vi "USB2XXXSPIADS1256.vi"() -> ()   [LabVIEW 2010]
uses:
  PublicFiles/usb_device/USB2XXX.dll
panel:
  out "mVp-p":dbl
  out "DC":dbl
  out "RMS":dbl
  out "Waveform Chart":dbl(graph)
  in  "pConfig":T1
  in  "Channel Index":i32(ring) items=["SPI1_CS0", "SPI2_CS0"]
  in  "Device Index":i32(ring) items=["0", "1", "2", "3", "4", "5"]
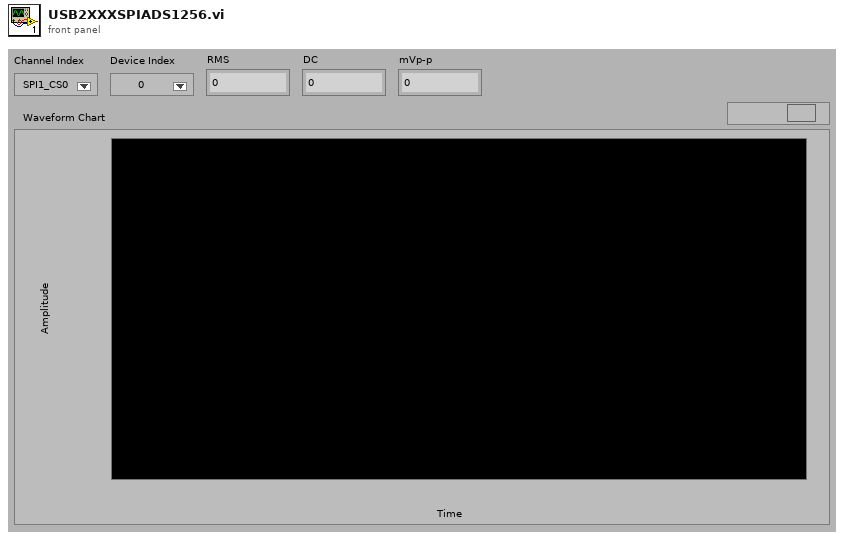
[diagram p1: front panel]
types:
  T1 = cluster{"Mode":i8, "Master":i8, "CPOL":i8, "CPHA":i8, "LSBFirst":i8, "SelPolarity":i8, "@dummy control@":i8, "@dummy control@":i8, "ClockSpeedHz":u32}
  T2 = enum16{"Init ADS1256", "Init SPI", "Read Data", "Close"}
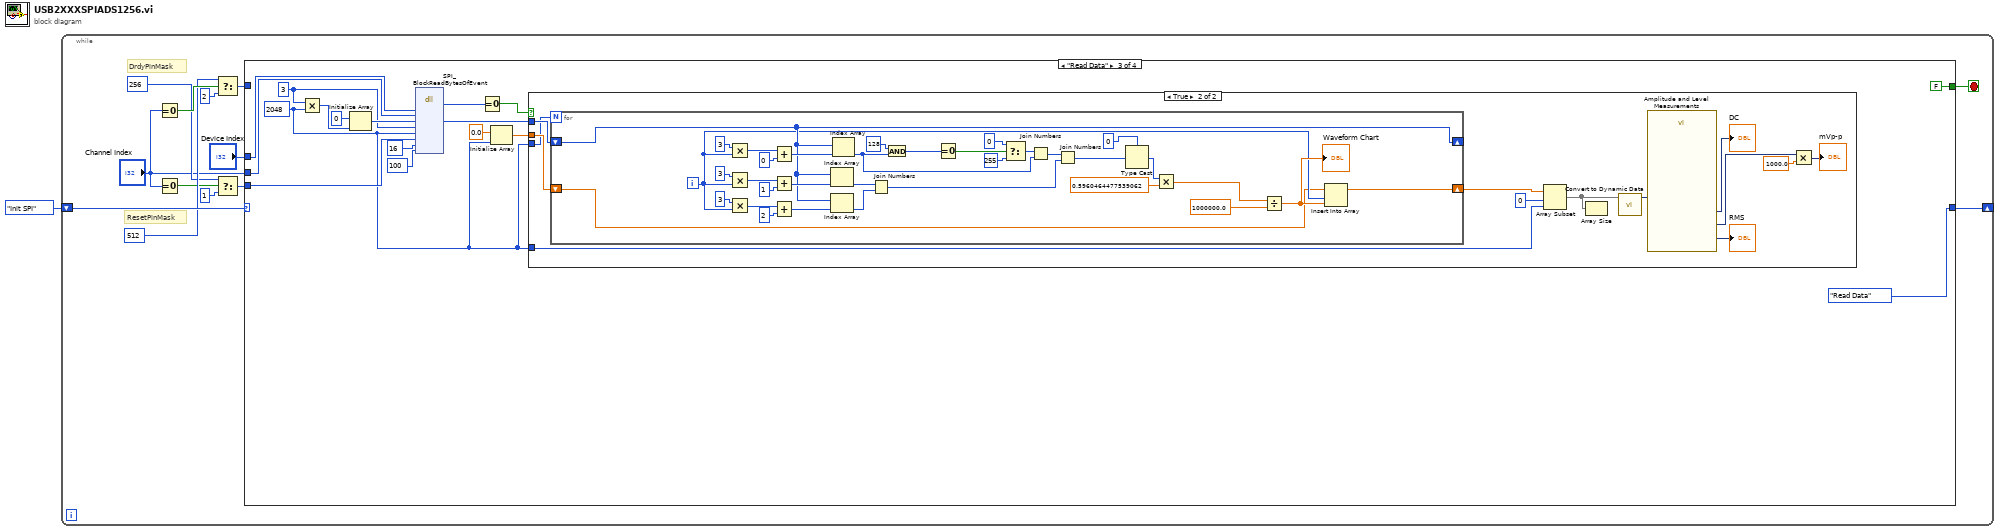
[diagram p0: block diagram]
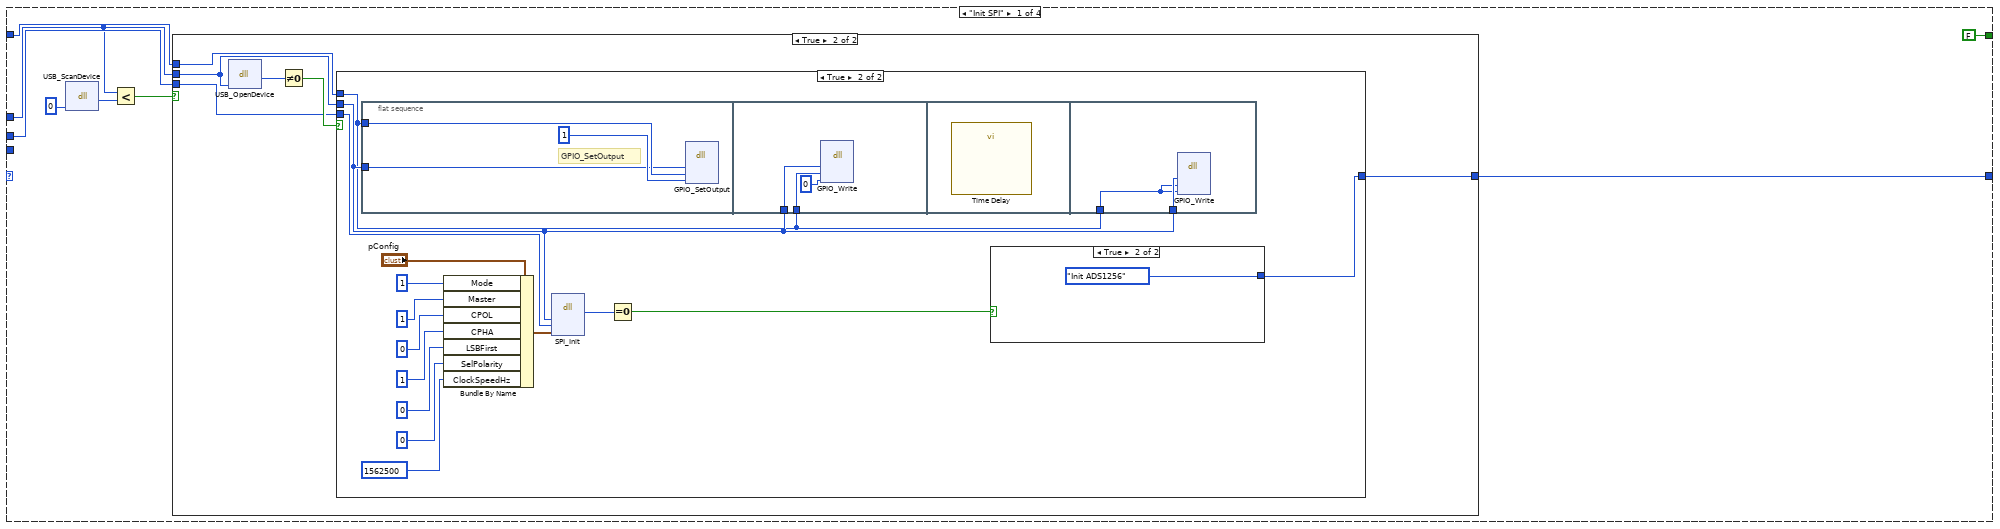
[diagram p2: hidden frame]
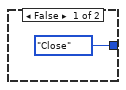
[diagram p3: hidden frame]
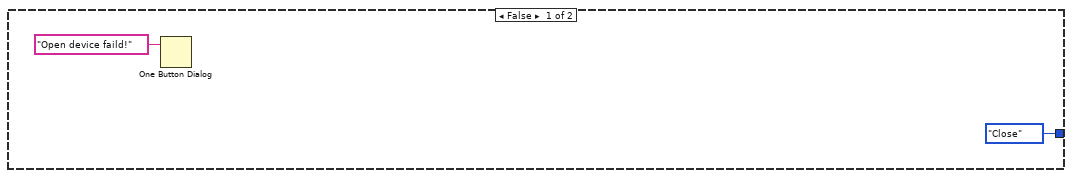
[diagram p4: hidden frame]
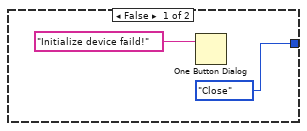
[diagram p5: hidden frame]
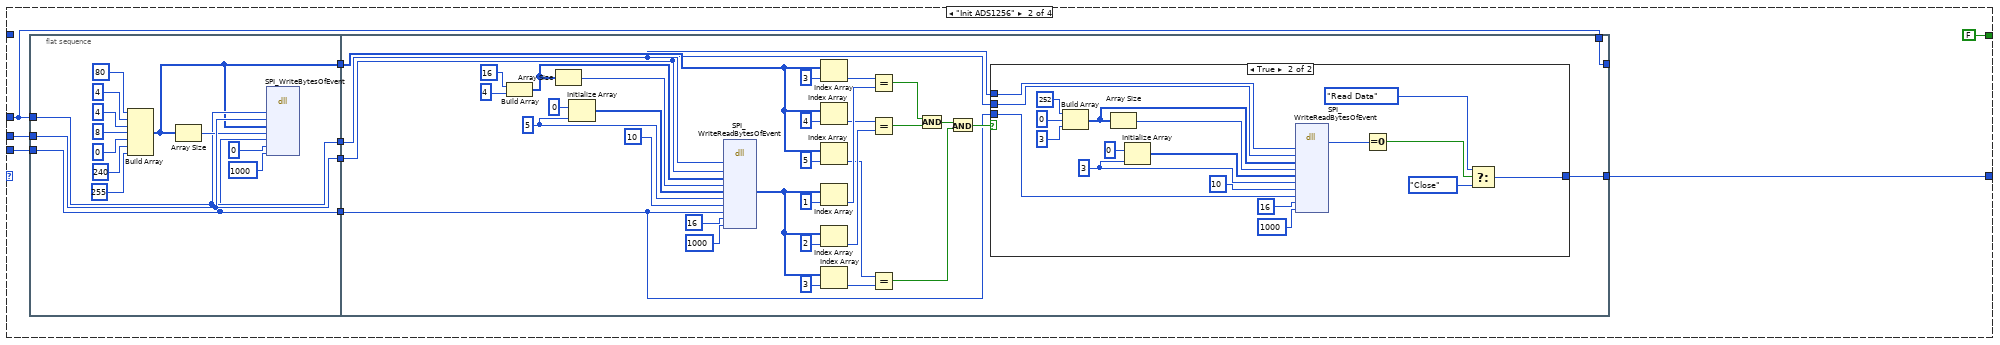
[diagram p6: hidden frame]
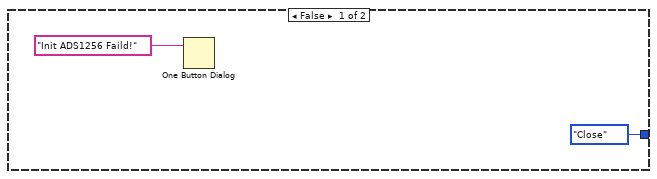
[diagram p7: hidden frame]
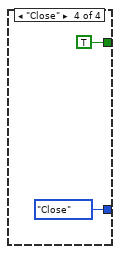
[diagram p9: hidden frame]
diagram:
  n1 = while {
    shift-right: [w13] -> _
    shift-left: T2."Init SPI" ("Enum") -> [w14]
    stop <- w11 stop-if-true
    # "DrdyPinMask"
    # "ResetPinMask"
    n2 = Equal To 0?(x="Channel Index") -> (x = 0?=w10:bool)
    n3 = Equal To 0?(x="Channel Index") -> (x = 0?=w7:bool)
    n4 = Select(t=u32 512 ("SelPolarity"), s=w10, f=u32 2 ("SelPolarity")) -> (s? t:f=w3:u32)
    n5 = Select(t=u32 256 ("SelPolarity"), s=w7, f=u32 1 ("SelPolarity")) -> (s? t:f=w2:u32)
    n6 = case shown="\"Read Data\"" w14 {
      tunnel: [w19 w58 T2."Read Data" ("Enum") T2."Close" ("Enum")] -> w13
      tunnel: "Device Index" -> [w16 w63 w149 _]
      tunnel: "Channel Index" -> [w18 w65 w148 _]
      tunnel: [FALSE FALSE FALSE TRUE] -> w11
      tunnel: w3 -> [w15 _ _ _]
      tunnel: w2 -> [_ w62 w144 _]
      frame "Init SPI" {
        n7 = dll-call lib="F:/OtherWork/STM32/USB2XXX_Example/trunk/Labview/PublicFiles/usb_device/USB2XXX.*" fn="USB_ScanDevice"("pDevNum"=0) -> (w21:i32)  [unwired: 4 in, 2 out]
        n8 = Less?(x=w16, y=w21) -> (x < y?=w20:bool)
        n9 = case shown="True" w20 {
          tunnel: w16 -> [_ w25]
          tunnel: w18 -> [_ w27]
          tunnel: [T2."Close" ("Enum") w26] -> w19
          tunnel: w15 -> [_ w24]
          frame False {
          }
          frame True {
            n10 = dll-call lib="F:/OtherWork/STM32/USB2XXX_Example/trunk/Labview/PublicFiles/usb_device/USB2XXX.*" fn="USB_OpenDevice"("DevIndex"=w25) -> (w29:u8)  [unwired: 4 in, 2 out]
            n11 = Not Equal To 0?(x=w29) -> (x != 0?=w28:bool)
            n12 = case shown="True" w28 {
              tunnel: w27 -> [_ w34]
              tunnel: w25 -> [_ w33]
              tunnel: [T2."Close" ("Enum") w45] -> w26
              tunnel: w24 -> [_ w32]
              frame False {
                n13 = One Button Dialog(message="Open device faild!") -> ()  [unwired: 1 in, 1 out]
              }
              frame True {
                n14 = flat-sequence {
                  tunnel: w32 -> [w48]
                  tunnel: w33 -> [w47]
                  tunnel: w33 -> [w52]
                  tunnel: w32 -> [w51]
                  tunnel: w33 -> [w54]
                  tunnel: w32 -> [w53]
                  frame #0 {
                    # "GPIO_SetOutput"
                    n15 = dll-call lib="F:/OtherWork/STM32/USB2XXX_Example/trunk/Labview/PublicFiles/usb_device/USB2XXX.*" fn="GPIO_SetOutput"("DevIndex"=w47, "PinMask"=w48, "PuPd"=u8 1) -> ()  [unwired: 7 in, 2 out]
                  }
                  frame #1 {
                    n16 = dll-call lib="F:/OtherWork/STM32/USB2XXX_Example/trunk/Labview/PublicFiles/usb_device/USB2XXX.*" fn="GPIO_Write"("DevIndex"=w52, "PinMask"=w51, "PinValue"=u32 0) -> ()  [unwired: 7 in, 2 out]
                  }
                  frame #2 {
                    n17 = call "Time Delay"() -> ()  [unwired: 11 in, 1 out]
                  }
                  frame #3 {
                    n18 = dll-call lib="F:/OtherWork/STM32/USB2XXX_Example/trunk/Labview/PublicFiles/usb_device/USB2XXX.*" fn="GPIO_Write"("DevIndex"=w54, "PinMask"=w53, "PinValue"=w53) -> ()  [unwired: 7 in, 2 out]
                  }
                }
                n19 = Bundle By Name(cluster="pConfig", "Mode"=i8 1, "Master"=i8 1, "CPOL"=i8 0, "CPHA"=i8 1, "LSBFirst"=i8 0, "SelPolarity"=i8 0, "ClockSpeedHz"=u32 1562500) -> (w44:T1)
                n20 = dll-call lib="F:/OtherWork/STM32/USB2XXX_Example/trunk/Labview/PublicFiles/usb_device/USB2XXX.*" fn="SPI_Init"("DevIndex"=w33, "SPIIndex"=w34, "pConfig"=w44) -> (w43:i32)  [unwired: 6 in, 2 out]
                n21 = Equal To 0?(x=w43) -> (x = 0?=w46:bool)
                n22 = case shown="True" w46 {
                  tunnel: [T2."Close" ("Enum") T2."Init ADS1256" ("Enum")] -> w45
                  frame False {
                    n23 = One Button Dialog(message="Initialize device faild!") -> ()  [unwired: 1 in, 1 out]
                  }
                  frame True {
                  }
                }
              }
            }
          }
        }
      }
      frame "Init ADS1256" {
        n24 = flat-sequence {
          tunnel: w63 -> [w69]
          tunnel: w65 -> [w73]
          tunnel: [w73] -> w64
          tunnel: w62 -> [w68]
          tunnel: [w69] -> w61
          tunnel: [w68] -> w60
          tunnel: [w67] -> w59
          tunnel: w64 -> [w82]
          tunnel: [w114] -> _
          tunnel: w63 -> [w114]
          tunnel: w61 -> [w83]
          tunnel: w60 -> [w81]
          tunnel: w59 -> [w96]
          tunnel: [w84] -> w58
          frame #0 {
            n25 = Build Array(u8 80, u8 4, u8 4, u8 8, u8 0, u8 240, u8 255) -> (w67:u8[])
            n26 = Array Size(array=w67) -> (size(s)=w72:i32)
            n27 = dll-call lib="F:/OtherWork/STM32/USB2XXX_Example/trunk/Labview/PublicFiles/usb_device/USB2XXX.*" fn="SPI_WriteBytesOfEvent"("DevIndex"=w69, "SPIIndex"=w73, "pWriteData"=w67, "WriteLen"=w72, "EventPin"=w68, "EventType"=u8 0, "TimeOutOfMs"=1000) -> ()  [unwired: 11 in, 2 out]
          }
          frame #1 {
            w107 = 5 ("dimension size")
            n28 = Build Array(u8 16, u8 4) -> (w110:u8[])
            n29 = Array Size(array=w110) -> (size(s)=w109:i32)
            n30 = Initialize Array(u8 0 ("element"), w107) -> (w108:u8[])
            n31 = dll-call lib="F:/OtherWork/STM32/USB2XXX_Example/trunk/Labview/PublicFiles/usb_device/USB2XXX.*" fn="SPI_WriteReadBytesOfEvent"("DevIndex"=w83, "SPIIndex"=w82, "pWriteData"=w110, "WriteLen"=w109, "pReadData"=w108, "ReadLen"=w107, "IntervalTimeUs"=10, "EventPin"=w81, "EventType"=u8 16, "TimeOutOfMs"=1000) -> ("pReadData"=w97:u8[])  [unwired: 13 in, 2 out]
            n32 = Index Array(array=w96, index=3) -> (element=w95:u8)
            n33 = Index Array(array=w96, index=4) -> (element=w93:u8)
            n34 = Index Array(array=w96, index=5) -> (element=w91:u8)
            n35 = Index Array(array=w97, index=1) -> (element=w94:u8)
            n36 = Index Array(array=w97, index=2) -> (element=w92:u8)
            n37 = Index Array(array=w97, index=3) -> (element=w90:u8)
            n38 = Equal?(x=w95, y=w94) -> (x = y?=w89:bool)
            n39 = Equal?(x=w93, y=w92) -> (x = y?=w88:bool)
            n40 = Equal?(x=w91, y=w90) -> (x = y?=w86:bool)
            n41 = And(x=w89, y=w88) -> (x .and. y?=w87:bool)
            n42 = And(x=w87, y=w86) -> (x .and. y?=w85:bool)
            n43 = case shown="True" w85 {
              tunnel: [T2."Close" ("Enum") w118] -> w84
              tunnel: w83 -> [_ w135]
              tunnel: w82 -> [_ w134]
              tunnel: w81 -> [_ w125]
              frame False {
                n44 = One Button Dialog(message="Init ADS1256 Faild!") -> ()  [unwired: 1 in, 1 out]
              }
              frame True {
                w117 = 3 ("dimension size")
                n45 = Build Array(u8 252, u8 0, u8 3) -> (w130:u8[])
                n46 = Array Size(array=w130) -> (size(s)=w129:i32)
                n47 = Initialize Array(u8 0 ("element"), w117) -> (w127:u8[])
                n48 = dll-call lib="F:/OtherWork/STM32/USB2XXX_Example/trunk/Labview/PublicFiles/usb_device/USB2XXX.*" fn="SPI_WriteReadBytesOfEvent"("DevIndex"=w135, "SPIIndex"=w134, "pWriteData"=w130, "WriteLen"=w129, "pReadData"=w127, "ReadLen"=w117, "IntervalTimeUs"=10, "EventPin"=w125, "EventType"=u8 16, "TimeOutOfMs"=1000) -> (w122:i32)  [unwired: 13 in, 2 out]
                n49 = Equal To 0?(x=w122) -> (x = 0?=w121:bool)
                n50 = Select(t=T2."Read Data" ("Enum"), s=w121, f=T2."Close" ("Enum")) -> (s? t:f=w118:T2)
              }
            }
          }
        }
      }
      frame "Read Data" {
        w136 = 2048 ("element")
        w145 = 3 ("element")
        n51 = Multiply(x=w145, y=w136) -> (x*y=w147:i32)
        n52 = Initialize Array(u8 0 ("element"), w147) -> (w146:u8[])
        n53 = dll-call lib="F:/OtherWork/STM32/USB2XXX_Example/trunk/Labview/PublicFiles/usb_device/USB2XXX.*" fn="SPI_BlockReadBytesOfEvent"("DevIndex"=w149, "SPIIndex"=w148, "pReadData"=w146, "BlockSize"=w145, "BlockNum"=w136, "EventPin"=w144, "EventType"=u8 16, "TimeOutOfMs"=100 ("TimeOutMs")) -> (w141:i32, "pReadData"=w139:u8[])  [unwired: 10 in, 2 out]
        n54 = Equal To 0?(x=w141) -> (x = 0?=w140:bool)
        n55 = Initialize Array(0.0 ("element"), w136) -> (w137:dbl[])
        n56 = case shown="True" w140 {
          tunnel: w136 -> [_ w160]
          tunnel: w139 -> [_ w165]
          tunnel: w137 -> [_ w161]
          tunnel: w136 -> [_ w156]
          frame False {
          }
          frame True {
            n57 = for {
              N: w160 -> [_]
              shift-right: [w170] -> _
              shift-left: w165 -> [w170]
              shift-right: [w166] -> w159
              shift-left: w161 -> [w167]
              i -> [w168]
              n58 = Multiply(x=3 ("element"), y=w168) -> (x*y=w198:i32)
              n59 = Multiply(x=3 ("element"), y=w168) -> (x*y=w193:i32)
              n60 = Multiply(x=3 ("element"), y=w168) -> (x*y=w190:i32)
              n61 = Add(x=w198, y=0) -> (x+y=w196:i32)
              n62 = Add(x=w193, y=1) -> (x+y=w195:i32)
              n63 = Add(x=w190, y=2) -> (x+y=w188:i32)
              n64 = Index Array(array=w170, index=w195) -> (element=w186:u8)
              n65 = Index Array(array=w170, index=w188) -> (element=w187:u8)
              n66 = Index Array(array=w170, index=w196) -> (element=w185:u8)
              n67 = Join Numbers(hi=w186, lo=w187) -> ((hi.lo)=w177:u16)
              n68 = And(x=u8 128 ("element"), y=w185) -> (x .and. y?=w182:u8)
              n69 = Equal To 0?(x=w182) -> (x = 0?=w183:bool)
              n70 = Select(t=u8 0 ("element"), s=w183, f=u8 255 ("element")) -> (s? t:f=w179:u8)
              n71 = Join Numbers(hi=w179, lo=w185) -> ((hi.lo)=w178:u16)
              n72 = Join Numbers(hi=w178, lo=w177) -> ((hi.lo)=w176:u32)
              n73 = Type Cast(type=0 ("element"), x=w176) -> (*(type *) &x=w174:i32)
              n74 = Multiply(x=w174, y=0.5960464477539062) -> (x*y=w172:dbl)
              n75 = Divide(x=w172, y=1000000.0) -> (x/y=w169:dbl)
              "Waveform Chart" <- w169
              n76 = Insert Into Array(array=w167, index=w168, new element=w169) -> (w166:dbl[])
            }
            n77 = Array Subset(array=w159, index=0, length=w156) -> (w158:dbl[])
            n78 = Array Size(array=w158) -> ()  [unwired: 1 out]
            n79 = call "Convert to Dynamic Data"("Array"=w158) -> ("Dynamic Data Type"=w164:dynamicdata)  [unwired: 3 in]
            n80 = call "Amplitude and Level Measurements"("Signals"=w164) -> ("Mean (DC)"=→"DC":dynamicdata, "RMS"=→"RMS":dynamicdata, "Peak to Peak"=w155:dynamicdata)  [unwired: 11 in, 1 out]
            n81 = Multiply(x=w155, y=1000.0) -> (x*y=→"mVp-p":dynamicdata)
          }
        }
      }
      frame "Close" {
      }
    }
  }
